vi "Move.vi"(8 "error in (no error)":errorcluster, 9 "Absolute (T)":bool=TRUE, 10 "Point":refnum<class "Point.lvclass">, 11 "IMovable in":refnum<class "IMovable.lvclass">) -> (0 "error out":errorcluster, 3 "IMovable out":refnum<class "IMovable.lvclass">)   [LabVIEW 2021, in "Picture2D.lvlib" / "IMovable.lvclass"]
uses:
  IMovable.lvclass
  Point/Point.lvclass
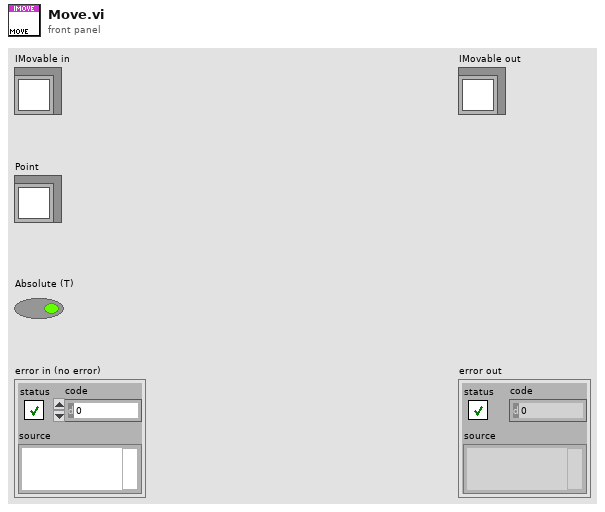
[diagram p1: front panel]
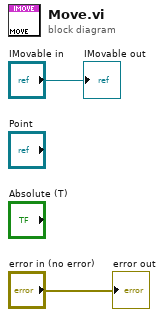
[diagram p0: block diagram]
diagram:
  "error out" <- "error in (no error)"
  "IMovable out" <- "IMovable in"
